vi "Fix Specific Errors.vi"(8 "error in (no error)":errorcluster, 9 "Good (reference) Node":refnum<k20>, 10 "Node to Fix":refnum<k20>, 11 "DOM document":refnum<k20>) -> (0 "error out":errorcluster, 2 "Node to Fix out":refnum<k20>)   [LabVIEW 2013]
uses:
  <vilib>/xml/Close Reference(Node).vi
  <vilib>/xml/NI_XML.lvlib
  <resource>/objmgr/DOMUserDefRef.rc
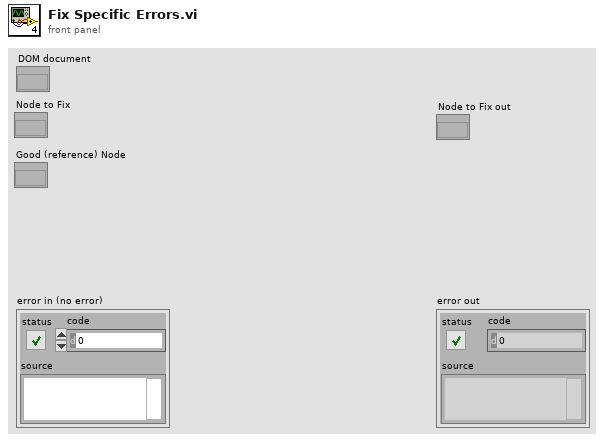
[diagram p1: front panel]
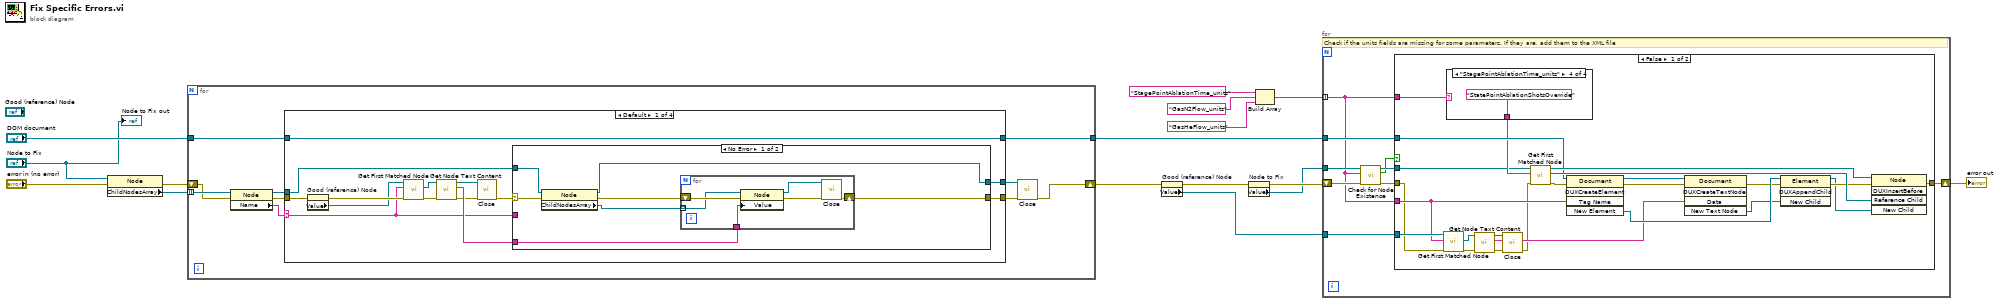
[diagram p0: block diagram]
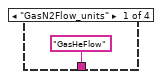
[diagram p2: hidden frame]
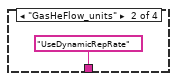
[diagram p3: hidden frame]
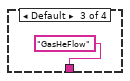
[diagram p4: hidden frame]
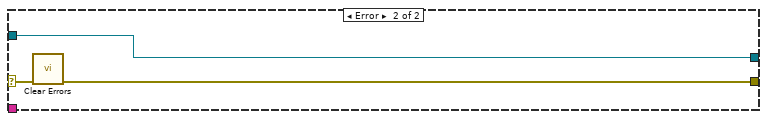
[diagram p6: hidden frame]
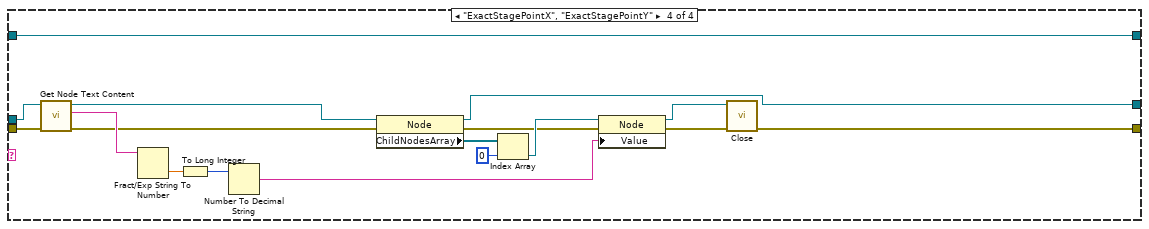
[diagram p9: hidden frame]
diagram:
  n1 = property class="Node"(reference="Node to Fix", error in="error in (no error)") -> (error out=w15:errorcluster, "ChildNodesArray"=w16:refnum<k20>[])  [unwired: 1 out]
  n2 = for {
    tunnel: w16 -> [w26] mode=indexing
    shift-right: [w19] -> w6
    shift-left: w15 -> [w22]
    tunnel: "DOM document" -> [w18]
    tunnel: [w17] -> w9
    n3 = property class="Node"(reference=w26, error in=w22) -> (reference out=w24:refnum<k20>, error out=w23:errorcluster, "Name"=w25:string)
    n4 = case shown="Default" w25 {
      selector: w25 -> [w32 _ _ _]
      tunnel: w24 -> [w39 w58 w60 w78]
      tunnel: w23 -> [w35 w59 w62 w79]
      tunnel: [w40 w59 w62 w63] -> w21
      tunnel: [w31 w58 w60 w66] -> w20
      tunnel: w18 -> [w27 w57 w61 w65]
      tunnel: [w27 w57 w61 w65] -> w17
      frame Default {
        n5 = property on="Good (reference) Node" class="XML Parser (strict)"(error in=w35) -> (error out=w34:errorcluster, "Value"=w33:refnum<k20>)  [unwired: 1 in, 1 out]
        n6 = call <vilib>:"Get First Matched Node.vi"("error in (no error)"=w34, "XPath expression"=w32, "node in"=w33) -> ("error out"=w37:errorcluster, "node result"=w38:refnum<k20>)  [unwired: 6 in, 1 out]
        n7 = call <vilib>:"Get Node Text Content.vi"("error in (no error)"=w37, "node in"=w38) -> ("error out"=w30:errorcluster, "node text"=w36:string, "node out"=w29:refnum<k20>)  [unwired: 7 in]
        n8 = call-poly <vilib>:"Close.vi"("error in (no error)"=w30, "node"=w29) -> ("error out"=w28:errorcluster)  [unwired: 7 in]
        n9 = case shown="No Error" w28 {
          selector: w28 -> [w46 w55]
          tunnel: [w43 w54] -> w40
          tunnel: w39 -> [w45 w56]
          tunnel: w36 -> [w47 _]
          tunnel: w32 -> [_ _]
          tunnel: [w44 w56] -> w31
          frame No Error {
            n10 = property class="Node"(reference=w45, error in=w46) -> (reference out=w44:refnum<k20>, error out=w42:errorcluster, "ChildNodesArray"=w41:refnum<k20>[])
            n11 = for {
              tunnel: w47 -> [w53]
              shift-right: [w50] -> w43
              shift-left: w42 -> [w49]
              tunnel: w41 -> [w48] mode=indexing
              n12 = property class="Node"(reference=w48, error in=w49, "Value"=w53) -> (reference out=w51:refnum<k20>, error out=w52:errorcluster)
              n13 = call-poly <vilib>:"Close.vi"("error in (no error)"=w52, "node"=w51) -> ("error out"=w50:errorcluster)  [unwired: 7 in]
            }
          }
          frame Error {
            n14 = call <vilib>:"Clear Errors.vi"("error in (no error)"=w55) -> ("error out"=w54:errorcluster)  [unwired: 6 in]
          }
        }
      }
      frame "AutoNumberTag", "DelaySettings", "SequenceNote", "TimingSettings" {
      }
      frame "#text", "Comment", "StagePointX", "StagePointY" {
      }
      frame "ExactStagePointX", "ExactStagePointY" {
        n15 = call <vilib>:"Get Node Text Content.vi"("error in (no error)"=w79, "node in"=w78) -> ("error out"=w68:errorcluster, "node text"=w75:string, "node out"=w67:refnum<k20>)  [unwired: 7 in]
        n16 = Fract/Exp String To Number(string=w75) -> (number=w77:dbl)  [unwired: 3 in, 1 out]
        n17 = To Long Integer(number=w77) -> (32bit integer=w76:i32)
        n18 = Number To Decimal String(number=w76) -> (decimal integer string=w64:string)  [unwired: 1 in]
        n19 = property class="Node"(reference=w67, error in=w68) -> (reference out=w66:refnum<k20>, error out=w71:errorcluster, "ChildNodesArray"=w74:refnum<k20>[])
        n20 = Index Array(array=w74, index=0) -> (element=w72:refnum<k20>)
        n21 = property class="Node"(reference=w72, error in=w71, "Value"=w64) -> (reference out=w69:refnum<k20>, error out=w70:errorcluster)
        n22 = call-poly <vilib>:"Close.vi"("error in (no error)"=w70, "node"=w69) -> ("error out"=w63:errorcluster)  [unwired: 7 in]
      }
    }
    n23 = call-poly <vilib>:"Close.vi"("error in (no error)"=w21, "node"=w20) -> ("error out"=w19:errorcluster)  [unwired: 7 in]
  }
  n24 = property on="Good (reference) Node" class="XML Parser (strict)"(error in=w6) -> (error out=w5:errorcluster, "Value"=w10:refnum<k20>)  [unwired: 1 in, 1 out]
  n25 = property on="Node to Fix" class="XML Parser (strict)"(error in=w5) -> (error out=w4:errorcluster, "Value"=w3:refnum<k20>)  [unwired: 1 in, 1 out]
  n26 = Build Array("StagePointAblationTime_units" ("XPath expression"), "GasN2Flow_units" ("XPath expression"), "GasHeFlow_units" ("XPath expression")) -> (w7:string[])
  n27 = for {
    tunnel: w3 -> [w83]
    tunnel: w10 -> [w88]
    tunnel: w9 -> [w87]
    tunnel: w7 -> [w80] mode=indexing
    shift-right: [w86] -> w8
    shift-left: w4 -> [w85]
    # "Check if the units fields are missing for some parameters. If they are, add them to the XML file"
    n28 = call "Check for Node Existence.vi"("error in (no error)"=w85, "XPath Expression"=w80, "Node to Search"=w83) -> ("error out"=w84:errorcluster, "Exists?"=w81:bool, "Node to Search out"=w82:refnum<k20>)  [unwired: 6 in]
    n29 = case shown="False" w81 {
      tunnel: w82 -> [w89 _]
      tunnel: w88 -> [w106 _]
      tunnel: w87 -> [w99 _]
      tunnel: [w98 w117] -> w86
      tunnel: w80 -> [w97 _]
      tunnel: w84 -> [w93 w117]
      tunnel: w80 -> [w95 _]
      frame False {
        n30 = call <vilib>:"Get First Matched Node.vi"("error in (no error)"=w93, "XPath expression"=w97, "node in"=w106) -> ("error out"=w94:errorcluster, "node result"=w105:refnum<k20>)  [unwired: 6 in, 1 out]
        n31 = case shown="\"StagePointAblationTime_units\"" w95 {
          tunnel: ["GasHeFlow" ("XPath expression") "UseDynamicRepRate" ("XPath expression") "GasHeFlow" ("XPath expression") "StatePointAblationShotsOverride" ("XPath expression")] -> w96
          frame "GasN2Flow_units" {
          }
          frame "GasHeFlow_units" {
          }
          frame Default {
          }
          frame "StagePointAblationTime_units" {
          }
        }
        n32 = call <vilib>:"Get Node Text Content.vi"("error in (no error)"=w94, "node in"=w105) -> ("error out"=w92:errorcluster, "node text"=w104:string, "node out"=w91:refnum<k20>)  [unwired: 7 in]
        n33 = call-poly <vilib>:"Close.vi"("error in (no error)"=w92, "node"=w91) -> ("error out"=w90:errorcluster)  [unwired: 7 in]
        n34 = call <vilib>:"Get First Matched Node.vi"("error in (no error)"=w90, "XPath expression"=w96, "node in"=w89) -> ("error out"=w107:errorcluster, "node result"=w102:refnum<k20>, "node out"=w103:refnum<k20>)  [unwired: 6 in]
        n35 = invoke class="Document" method="DUXCreateElement"(reference=w99, error in=w107, "Tag Name"=w97) -> (reference out=w108:refnum<k20>, error out=w109:errorcluster, "New Element"=w112:refnum<k20>)  [unwired: 2 in, 2 out]
        n36 = invoke class="Document" method="DUXCreateTextNode"(reference=w108, error in=w109, "Data"=w104) -> (error out=w110:errorcluster, "New Text Node"=w111:refnum<k20>)  [unwired: 2 in, 3 out]
        n37 = invoke class="Element" method="DUXAppendChild"(reference=w112, error in=w110, "New Child"=w111) -> (reference out=w100:refnum<k20>, error out=w101:errorcluster)  [unwired: 1 in, 2 out]
        n38 = invoke class="Node" method="DUXInsertBefore"(reference=w103, error in=w101, "Reference Child"=w102, "New Child"=w100) -> (error out=w98:errorcluster)  [unwired: 1 in, 4 out]
      }
      frame True {
      }
    }
  }
  "error out" <- w8
  "Node to Fix out" <- "Node to Fix"
